vi "EXP1 TIME.vi"(8 "s 2":bool, 9 "s":bool, 10 "s 4":bool, 11 "s 3":bool) -> (0 "time 2":i32, 1 "time":i32, 2 "time 4":i32, 3 "time 3":i32)   [LabVIEW 2018]
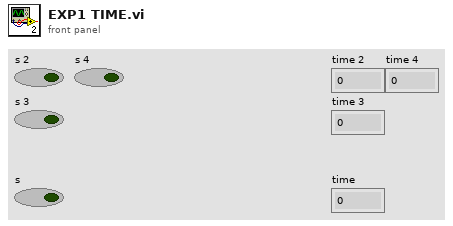
[diagram p1: front panel]
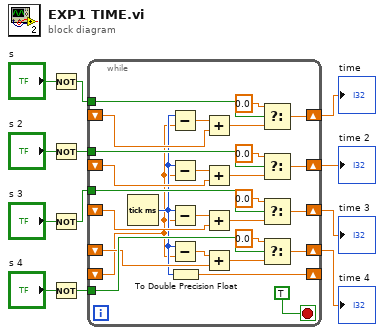
[diagram p0: block diagram]
diagram:
  n1 = Not(x="s") -> (.not. x?=w10:bool)
  n2 = Not(x="s 2") -> (.not. x?=w6:bool)
  n3 = Not(x="s 3") -> (.not. x?=w5:bool)
  n4 = Not(x="s 4") -> (.not. x?=w4:bool)
  n5 = while {
    shift-right: [w27] -> w12
    shift-left: _ -> [w39]
    shift-right: [w37] -> _
    shift-left: _ -> [w13]
    tunnel: w10 -> [w35]
    tunnel: w6 -> [w31]
    tunnel: w5 -> [w30]
    tunnel: w4 -> [w29]
    shift-right: [w26] -> w3
    shift-left: _ -> [w20]
    shift-right: [w25] -> w2
    shift-left: _ -> [w18]
    shift-right: [w24] -> w1
    shift-left: _ -> [w16]
    stop <- TRUE stop-if-true
    n6 = Tick Count (ms)() -> (millisecond timer value=w14:u32)
    n7 = Subtract(x=w14, y=w13) -> (x-y=w40:dbl)
    n8 = Subtract(x=w14, y=w13) -> (x-y=w21:dbl)
    n9 = Subtract(x=w14, y=w13) -> (x-y=w23:dbl)
    n10 = Subtract(x=w14, y=w13) -> (x-y=w22:dbl)
    n11 = To Double Precision Float(number=w14) -> (double precision float=w37:dbl)
    n12 = Add(x=w40, y=w39) -> (x+y=w28:dbl)
    n13 = Add(x=w21, y=w20) -> (x+y=w19:dbl)
    n14 = Add(x=w23, y=w18) -> (x+y=w17:dbl)
    n15 = Add(x=w22, y=w16) -> (x+y=w15:dbl)
    n16 = Select(t=0.0, s=w35, f=w28) -> (s? t:f=w27:dbl)
    n17 = Select(t=0.0, s=w31, f=w19) -> (s? t:f=w26:dbl)
    n18 = Select(t=0.0, s=w30, f=w17) -> (s? t:f=w25:dbl)
    n19 = Select(t=0.0, s=w29, f=w15) -> (s? t:f=w24:dbl)
  }
  "time" <- w12
  "time 2" <- w3
  "time 3" <- w2
  "time 4" <- w1
